vi "Enqueue User Que.vi"   [LabVIEW 2016]
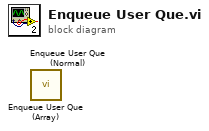
[diagram p0: block diagram]
diagram:
  n1 = call "Enqueue User Que (Array).vi"() -> ()  [unwired: 9 in, 3 out]
  n2 = call "Enqueue User Que (Normal).vi"() -> ()  [unwired: 9 in, 3 out]
